vi "2Decembre2016.vi"() -> ()   [LabVIEW 2014]
panel:
  out "Combinaison 2":i8[](array[numeric])
  out "Chiffre 2":i8 format="%x"
  out "Combinaison":i8[](array[numeric])
  out "Chiffre":i8
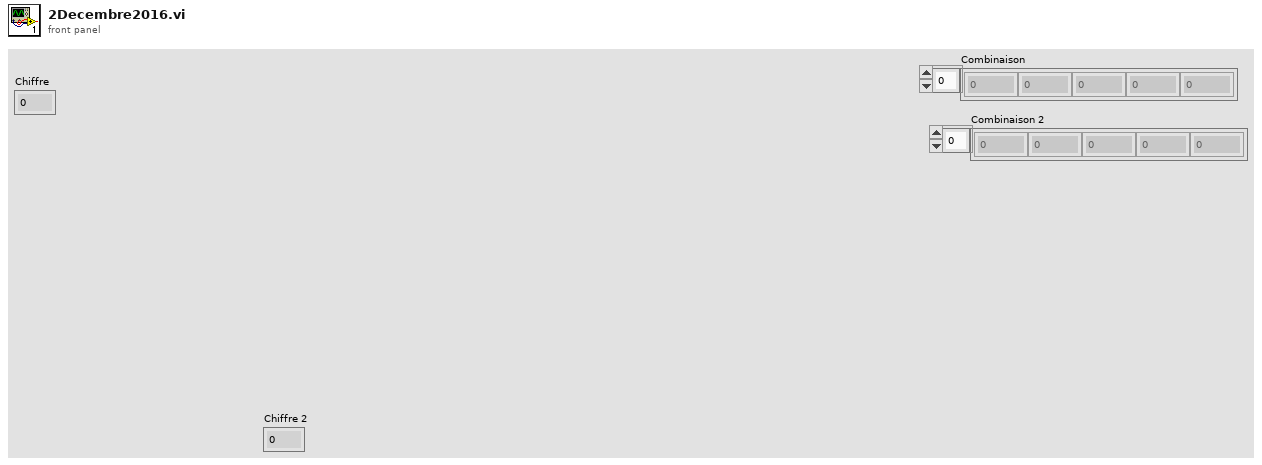
[diagram p1: front panel]
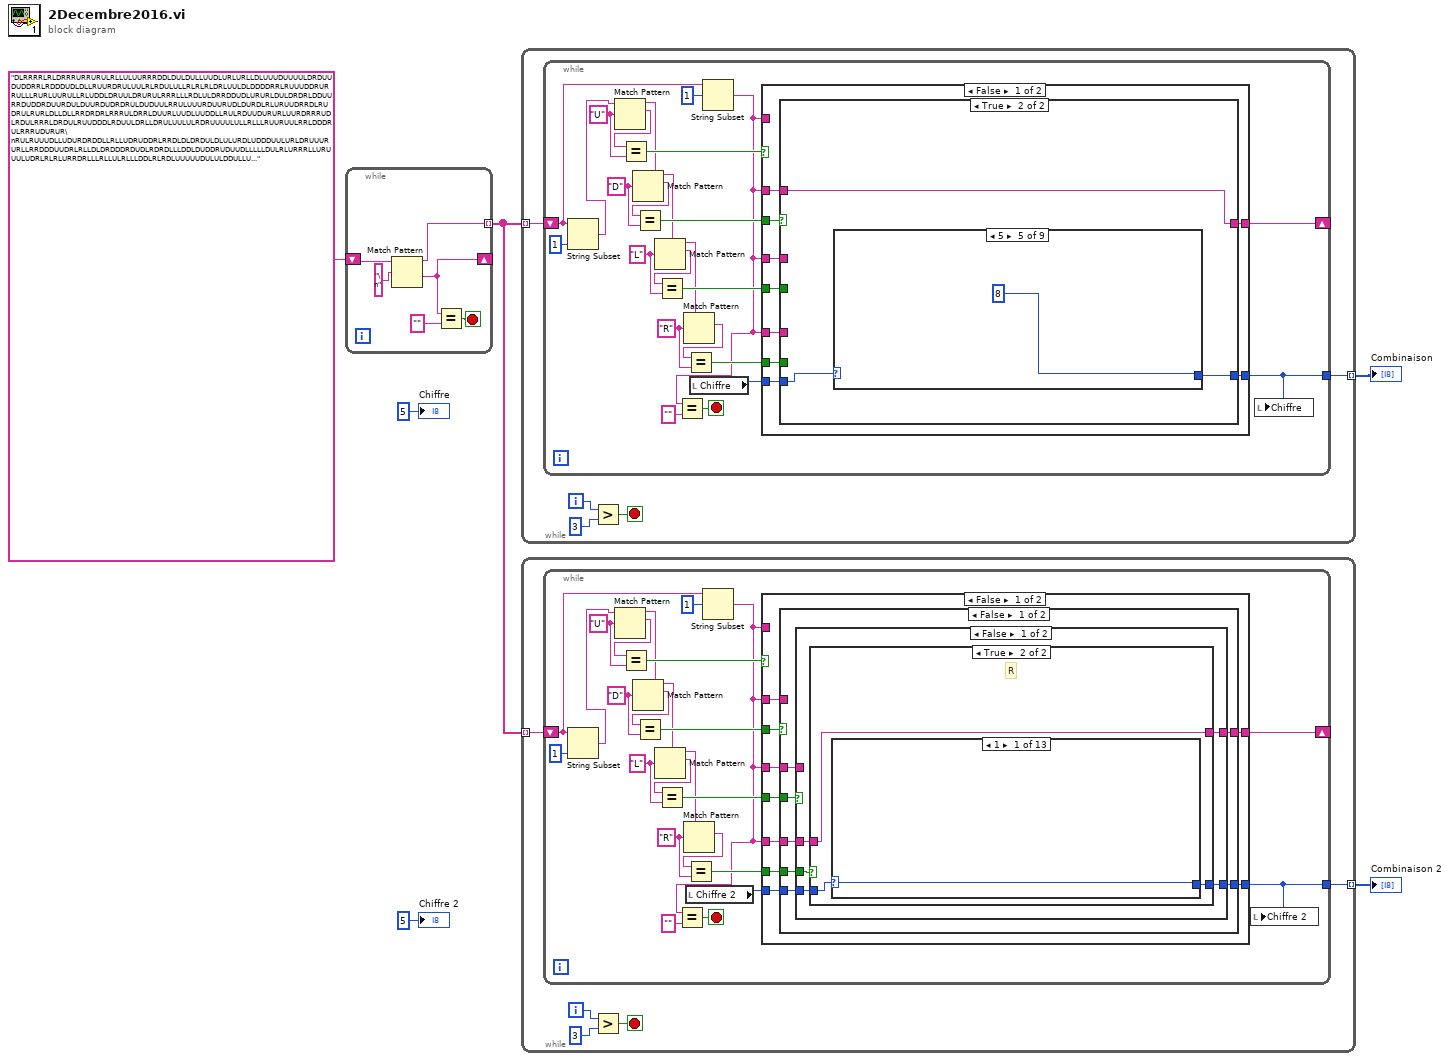
[diagram p0: block diagram]
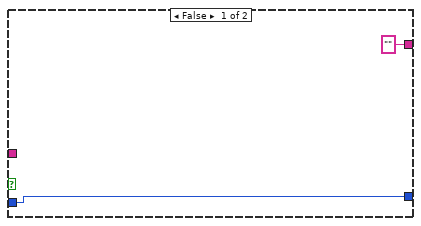
[diagram p2: hidden frame]
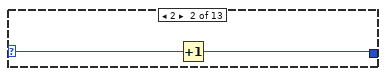
[diagram p3: hidden frame]
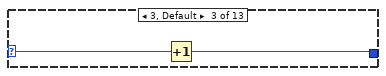
[diagram p4: hidden frame]
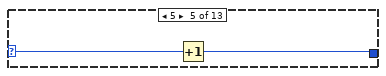
[diagram p6: hidden frame]
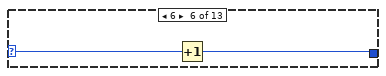
[diagram p7: hidden frame]
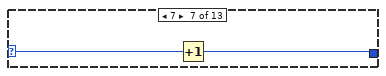
[diagram p8: hidden frame]
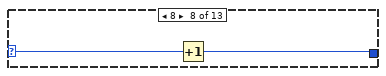
[diagram p9: hidden frame]
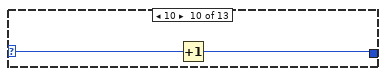
[diagram p11: hidden frame]
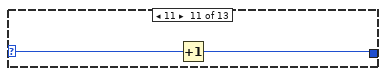
[diagram p12: hidden frame]
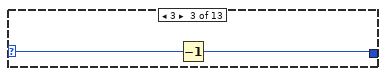
[diagram p17: hidden frame]
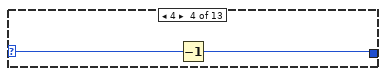
[diagram p18: hidden frame]
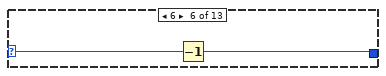
[diagram p20: hidden frame]
diagram:
  n1 = while {
    shift-right: [w9] -> _
    shift-left: "DLRRRRLRLDRRRURRURULRLLULUURRRDDLDULDULLUUDLURLURLLDLUUUDUUUULDRDUUDUDDRRLRDDDUDLDLLRUURDRULUULRLRDULULLRLRLRLDRLUULDLDDDDRRLRUUUDDRURRULLLRURLUURULLRLUDDLDRUULDRURULRRRLLLRDLULDRRDDUDLURURLDULDRDRLDDUURRDUDDRDUURDULDUURDUDRDRULDUDUULRRULUUURDUURUDLDURDLRLURUUDRRDLRUDRULRURLDLLDLLRRDRDRLRRRULDRRLDUURLUUDLUUDDLLRULRDUUDURURLUURDRRRUDLRDULRRRLDRDULRUUDDDLRDUULDRLLDRULUULULRDRUUUULULLRLLLRUURUULRRLDDDRULRRRUDURUR\nRULRUUUDLLUDURDRDDLLRLLUDRUDDRLRRDLDLDRDULDLULURDLUDDDUULURLDRUUURURLLRRDDDUUDRLRLLDLDRDDDRDUDLRDRDLLLDDLDUDDRUDUUDLLLLLDULRLURRRLLURUUULUDRLRLRLURRDRLLLRLLULRLLLDDLRLRDLUUUUUDULULDDULLU..." -> [w12]
    tunnel: [w11] -> w1 mode=indexing
    stop <- w10 stop-if-true
    n2 = Match Pattern(string=w12, regular expression="\n") -> (before substring=w11:string, after substring=w9:string)  [unwired: 1 in, 2 out]
    n3 = Equal?(x=w9, y="") -> (x = y?=w10:bool)
  }
  n4 = while {
    tunnel: w1 -> [w13] mode=indexing
    tunnel: [w14] -> w5 mode=indexing
    i -> [w16]
    stop <- w15 stop-if-true
    n5 = while {
      shift-right: [w33] -> _
      shift-left: w13 -> [w23]
      tunnel: [w26] -> w14
      stop <- w28 stop-if-true
      w35 = "R"
      w37 = "L"
      w39 = "D"
      w41 = "U"
      n6 = String Subset(string=w23, length (rest)=1 ("length (rest)")) -> (substring=w24:string)  [unwired: 1 in]
      n7 = Match Pattern(string=w24, regular expression=w41) -> (before substring=w21:string, match substring=w42:string)  [unwired: 1 in, 2 out]
      n8 = Equal?(x=w42, y=w41) -> (x = y?=w34:bool)
      n9 = Match Pattern(string=w21, regular expression=w39) -> (before substring=w20:string, match substring=w40:string)  [unwired: 1 in, 2 out]
      n10 = Equal?(x=w40, y=w39) -> (x = y?=w32:bool)
      n11 = Match Pattern(string=w20, regular expression=w37) -> (before substring=w19:string, match substring=w38:string)  [unwired: 1 in, 2 out]
      n12 = Equal?(x=w38, y=w37) -> (x = y?=w31:bool)
      n13 = Match Pattern(string=w19, regular expression=w35) -> (match substring=w36:string)  [unwired: 1 in, 3 out]
      n14 = Equal?(x=w36, y=w35) -> (x = y?=w30:bool)
      n15 = local read "Chiffre"() -> (w27:i8)
      n16 = String Subset(string=w23, offset (0)=1) -> (substring=w18:string)  [unwired: 1 in]
      n17 = Equal?(x=w18, y="") -> (x = y?=w28:bool)
      n18 = case shown="False" w34 {
        tunnel: [w47 w116] -> w33
        tunnel: w32 -> [w51 _]
        tunnel: w18 -> [_ w116]
        tunnel: w18 -> [w50 _]
        tunnel: w18 -> [w49 _]
        tunnel: w18 -> [w48 _]
        tunnel: w31 -> [w46 _]
        tunnel: w30 -> [w45 _]
        tunnel: w27 -> [w44 w114]
        tunnel: [w43 w115] -> w26
        frame False {
          n19 = case shown="True" w51 {
            tunnel: w50 -> [_ w104]
            tunnel: w49 -> [w56 _]
            tunnel: w48 -> [w54 _]
            tunnel: [w57 w104] -> w47
            tunnel: w46 -> [w58 _]
            tunnel: w45 -> [w55 _]
            tunnel: w44 -> [w53 w102]
            tunnel: [w52 w103] -> w43
            frame False {
              n20 = case shown="False" w58 {
                tunnel: [w62 w86] -> w57
                tunnel: w56 -> [_ w86]
                tunnel: w55 -> [w63 _]
                tunnel: w54 -> [w61 _]
                tunnel: w53 -> [w60 w84]
                tunnel: [w59 w85] -> w52
                frame False {
                  n21 = case shown="False" w63 {
                    tunnel: ["" w68] -> w62
                    tunnel: w61 -> [_ w68]
                    tunnel: w60 -> [w64 w67]
                    tunnel: [w64 w66] -> w59
                    frame False {
                    }
                    frame True {
                      # "R"
                      n22 = case shown="9" w67 {
                        selector: w67 -> [w70 w72 w73 w75 w77 w78 w80 w82 w83]
                        tunnel: [w69 w71 w73 w74 w76 w78 w79 w81 w83] -> w66
                        frame 1 {
                          n23 = Increment(x=w70) -> (x+1=w69:i8)
                        }
                        frame 2 {
                          n24 = Increment(x=w72) -> (x+1=w71:i8)
                        }
                        frame 3, Default {
                        }
                        frame 4 {
                          n25 = Increment(x=w75) -> (x+1=w74:i8)
                        }
                        frame 5 {
                          n26 = Increment(x=w77) -> (x+1=w76:i8)
                        }
                        frame 6 {
                        }
                        frame 7 {
                          n27 = Increment(x=w80) -> (x+1=w79:i8)
                        }
                        frame 8 {
                          n28 = Increment(x=w82) -> (x+1=w81:i8)
                        }
                        frame 9 {
                        }
                      }
                    }
                  }
                }
                frame True {
                  n29 = case shown="9" w84 {
                    selector: w84 -> [w87 w89 w91 w92 w94 w96 w97 w99 w101]
                    tunnel: [w87 w88 w90 w92 w93 w95 w97 w98 w100] -> w85
                    frame 1, Default {
                    }
                    frame 2 {
                      n30 = Decrement(x=w89) -> (x-1=w88:i8)
                    }
                    frame 3 {
                      n31 = Decrement(x=w91) -> (x-1=w90:i8)
                    }
                    frame 4 {
                    }
                    frame 5 {
                      n32 = Decrement(x=w94) -> (x-1=w93:i8)
                    }
                    frame 6 {
                      n33 = Decrement(x=w96) -> (x-1=w95:i8)
                    }
                    frame 7 {
                    }
                    frame 8 {
                      n34 = Decrement(x=w99) -> (x-1=w98:i8)
                    }
                    frame 9 {
                      n35 = Decrement(x=w101) -> (x-1=w100:i8)
                    }
                  }
                }
              }
            }
            frame True {
              n36 = case shown="5" w102 {
                selector: w102 -> [_ _ _ _ _ _ w111 w112 w113]
                tunnel: [4 ("Chiffre") 5 ("Chiffre") 6 ("Chiffre") 7 ("Chiffre") 8 ("Chiffre") 9 ("Chiffre") w111 w112 w113] -> w103
                frame 1 {
                }
                frame 2 {
                }
                frame 3 {
                }
                frame 4 {
                }
                frame 5 {
                }
                frame 6 {
                }
                frame 7 {
                }
                frame 8 {
                }
                frame 9, Default {
                }
              }
            }
          }
        }
        frame True {
          n37 = case shown="5" w114 {
            selector: w114 -> [w117 w118 w119 _ _ _ _ _ _]
            tunnel: [w117 w118 w119 1 ("Chiffre") 2 ("Chiffre") 3 ("Chiffre") 4 ("Chiffre") 5 ("Chiffre") 6 ("Chiffre")] -> w115
            frame 1, Default {
            }
            frame 2 {
            }
            frame 3 {
            }
            frame 4 {
            }
            frame 5 {
            }
            frame 6 {
            }
            frame 7 {
            }
            frame 8 {
            }
            frame 9 {
            }
          }
        }
      }
      n38 = local write "Chiffre"(w26) -> ()
    }
    n39 = Greater?(x=w16, y=3) -> (0:w15:bool)
  }
  "Combinaison" <- w5
  n40 = while {
    tunnel: w1 -> [w126] mode=indexing
    tunnel: [w127] -> w3 mode=indexing
    i -> [w129]
    stop <- w128 stop-if-true
    n41 = while {
      shift-right: [w146] -> _
      shift-left: w126 -> [w136]
      tunnel: [w139] -> w127
      stop <- w141 stop-if-true
      w148 = "R"
      w150 = "L"
      w152 = "D"
      w154 = "U"
      n42 = String Subset(string=w136, length (rest)=1 ("length (rest)")) -> (substring=w137:string)  [unwired: 1 in]
      n43 = Match Pattern(string=w137, regular expression=w154) -> (before substring=w134:string, match substring=w155:string)  [unwired: 1 in, 2 out]
      n44 = Equal?(x=w155, y=w154) -> (x = y?=w147:bool)
      n45 = Match Pattern(string=w134, regular expression=w152) -> (before substring=w133:string, match substring=w153:string)  [unwired: 1 in, 2 out]
      n46 = Equal?(x=w153, y=w152) -> (x = y?=w145:bool)
      n47 = Match Pattern(string=w133, regular expression=w150) -> (before substring=w132:string, match substring=w151:string)  [unwired: 1 in, 2 out]
      n48 = Equal?(x=w151, y=w150) -> (x = y?=w144:bool)
      n49 = Match Pattern(string=w132, regular expression=w148) -> (match substring=w149:string)  [unwired: 1 in, 3 out]
      n50 = Equal?(x=w149, y=w148) -> (x = y?=w143:bool)
      n51 = local read "Chiffre 2"() -> (w140:i8)
      n52 = String Subset(string=w136, offset (0)=1) -> (substring=w131:string)  [unwired: 1 in]
      n53 = Equal?(x=w131, y="") -> (x = y?=w141:bool)
      n54 = case shown="False" w147 {
        tunnel: [w160 w245] -> w146
        tunnel: w145 -> [w164 _]
        tunnel: w131 -> [_ w245]
        tunnel: w131 -> [w163 _]
        tunnel: w131 -> [w162 _]
        tunnel: w131 -> [w161 _]
        tunnel: w144 -> [w159 _]
        tunnel: w143 -> [w158 _]
        tunnel: w140 -> [w157 w243]
        tunnel: [w156 w244] -> w139
        frame False {
          n55 = case shown="False" w164 {
            tunnel: w163 -> [_ w229]
            tunnel: w162 -> [w169 _]
            tunnel: w161 -> [w167 _]
            tunnel: [w170 w229] -> w160
            tunnel: w159 -> [w171 _]
            tunnel: w158 -> [w168 _]
            tunnel: w157 -> [w166 w227]
            tunnel: [w165 w228] -> w156
            frame False {
              n56 = case shown="False" w171 {
                tunnel: [w175 w205] -> w170
                tunnel: w169 -> [_ w205]
                tunnel: w168 -> [w176 _]
                tunnel: w167 -> [w174 _]
                tunnel: w166 -> [w173 w203]
                tunnel: [w172 w204] -> w165
                frame False {
                  n57 = case shown="True" w176 {
                    tunnel: ["" w181] -> w175
                    tunnel: w174 -> [_ w181]
                    tunnel: w173 -> [w177 w180]
                    tunnel: [w177 w179] -> w172
                    frame False {
                    }
                    frame True {
                      # "R"
                      n58 = case shown="1" w180 {
                        selector: w180 -> [w182 w184 w186 w187 w189 w191 w193 w195 w196 w198 w200 w201 w202]
                        tunnel: [w182 w183 w185 w187 w188 w190 w192 w194 w196 w197 w199 w201 w202] -> w179
                        frame 1 {
                        }
                        frame 2 {
                          n59 = Increment(x=w184) -> (x+1=w183:i8)
                        }
                        frame 3, Default {
                          n60 = Increment(x=w186) -> (x+1=w185:i8)
                        }
                        frame 4 {
                        }
                        frame 5 {
                          n61 = Increment(x=w189) -> (x+1=w188:i8)
                        }
                        frame 6 {
                          n62 = Increment(x=w191) -> (x+1=w190:i8)
                        }
                        frame 7 {
                          n63 = Increment(x=w193) -> (x+1=w192:i8)
                        }
                        frame 8 {
                          n64 = Increment(x=w195) -> (x+1=w194:i8)
                        }
                        frame 9 {
                        }
                        frame 10 {
                          n65 = Increment(x=w198) -> (x+1=w197:i8)
                        }
                        frame 11 {
                          n66 = Increment(x=w200) -> (x+1=w199:i8)
                        }
                        frame 12 {
                        }
                        frame 13 {
                        }
                      }
                    }
                  }
                }
                frame True {
                  n67 = case shown="2" w203 {
                    selector: w203 -> [w206 w207 w209 w211 w212 w214 w216 w218 w220 w221 w223 w225 w226]
                    tunnel: [w206 w207 w208 w210 w212 w213 w215 w217 w219 w221 w222 w224 w226] -> w204
                    frame 1, Default {
                    }
                    frame 2 {
                    }
                    frame 3 {
                      n68 = Decrement(x=w209) -> (x-1=w208:i8)
                    }
                    frame 4 {
                      n69 = Decrement(x=w211) -> (x-1=w210:i8)
                    }
                    frame 5 {
                    }
                    frame 6 {
                      n70 = Decrement(x=w214) -> (x-1=w213:i8)
                    }
                    frame 7 {
                      n71 = Decrement(x=w216) -> (x-1=w215:i8)
                    }
                    frame 8 {
                      n72 = Decrement(x=w218) -> (x-1=w217:i8)
                    }
                    frame 9 {
                      n73 = Decrement(x=w220) -> (x-1=w219:i8)
                    }
                    frame 10 {
                    }
                    frame 11 {
                      n74 = Decrement(x=w223) -> (x-1=w222:i8)
                    }
                    frame 12 {
                      n75 = Decrement(x=w225) -> (x-1=w224:i8)
                    }
                    frame 13 {
                    }
                  }
                }
              }
            }
            frame True {
              n76 = case shown="12" w227 {
                selector: w227 -> [_ _ _ _ w234 _ _ _ w238 w239 _ w241 w242]
                tunnel: [3 ("Chiffre") 6 ("Chiffre") 7 ("Chiffre") 8 ("Chiffre") w234 10 ("Chiffre") 11 ("Chiffre") 12 ("Chiffre") w238 w239 i8 13 ("Chiffre 2") w241 w242] -> w228
                frame 1 {
                }
                frame 2 {
                }
                frame 3 {
                }
                frame 4 {
                }
                frame 5 {
                }
                frame 6 {
                }
                frame 7 {
                }
                frame 8 {
                }
                frame 9, Default {
                }
                frame 10 {
                }
                frame 11 {
                }
                frame 12 {
                }
                frame 13 {
                }
              }
            }
          }
        }
        frame True {
          n77 = case shown="13" w243 {
            selector: w243 -> [w246 w247 _ w249 w250 _ _ _ w254 _ _ _ _]
            tunnel: [w246 w247 1 ("Chiffre") w249 w250 2 ("Chiffre") 3 ("Chiffre") 4 ("Chiffre") w254 i8 6 ("Chiffre 2") i8 7 ("Chiffre 2") i8 8 ("Chiffre 2") i8 11 ("Chiffre 2")] -> w244
            frame 1, Default {
            }
            frame 2 {
            }
            frame 3 {
            }
            frame 4 {
            }
            frame 5 {
            }
            frame 6 {
            }
            frame 7 {
            }
            frame 8 {
            }
            frame 9 {
            }
            frame 10 {
            }
            frame 11 {
            }
            frame 12 {
            }
            frame 13 {
            }
          }
        }
      }
      n78 = local write "Chiffre 2"(w139) -> ()
    }
    n79 = Greater?(x=w129, y=3) -> (0:w128:bool)
  }
  "Combinaison 2" <- w3
  "Chiffre" <- 5 ("Chiffre")
  "Chiffre 2" <- i8 5 ("Chiffre 2")
